vi "Header and Footer.vi"(4 "Header Footer Table Konfig":T8={"Header"={"Table Settings"={"Number of Columns"=2, "Width (%)"=100.0, "Relative Column Widths (%)"=[80.0, 20.0], "Horizontal Align"=0, "Header Rows"=0}, "Cell Defaults"={"Background Color"=16777215, "Horizontal Align"=3, "Vertical Align"=1, "Minimum Height"=0.0, "Fixed Height"=0.0, "Padding"={"Left"=2.0, "Top"=2.0, "Right"=2.0, "Bottom"=3.0}}, "Borders"={"Left"={"Enabled"=FALSE, "Width"=1.0, "Color"=0}, "Top"={"Enabled"=FALSE, "Width"=1.0, "Color"=0}, "Right"={"Enabled"=FALSE, "Width"=1.0, "Color"=0}, "Bottom"={"Enabled"=FALSE, "Width"=1.0, "Color"=0}, "Middle Horizontal"={"Enabled"=FALSE, "Width"=0.5, "Color"=0}, "Middle Vertical"={"Enabled"=FALSE, "Width"=0.5, "Color"=0}}}, "Footer"={"Table Settings"={"Number of Columns"=3, "Width (%)"=100.0, "Relative Column Widths (%)"=[15.0, 70.0, 15.0], "Horizontal Align"=0, "Header Rows"=0}, "Cell Defaults"={"Background Color"=16777215, "Horizontal Align"=0, "Vertical Align"=1, "Minimum Height"=0.0, "Fixed Height"=0.0, "Padding"={"Left"=2.0, "Top"=2.0, "Right"=2.0, "Bottom"=3.0}}, "Borders"={"Left"={"Enabled"=FALSE, "Width"=1.0, "Color"=0}, "Top"={"Enabled"=FALSE, "Width"=1.0, "Color"=0}, "Right"={"Enabled"=FALSE, "Width"=1.0, "Color"=0}, "Bottom"={"Enabled"=FALSE, "Width"=1.0, "Color"=0}, "Middle Horizontal"={"Enabled"=FALSE, "Width"=0.5, "Color"=0}, "Middle Vertical"={"Enabled"=FALSE, "Width"=0.5, "Color"=0}}}, "Footer Logo Row"={"Table Settings"={"Number of Columns"=1, "Width (%)"=100.0, "Relative Column Widths (%)"=[100.0], "Horizontal Align"=0, "Header Rows"=0}, "Cell Defaults"={"Background Color"=16777215, "Horizontal Align"=0, "Vertical Align"=1, "Minimum Height"=0.0, "Fixed Height"=0.0, "Padding"={"Left"=2.0, "Top"=2.0, "Right"=2.0, "Bottom"=3.0}}, "Borders"={"Left"={"Enabled"=FALSE, "Width"=1.0, "Color"=0}, "Top"={"Enabled"=FALSE, "Width"=1.0, "Color"=0}, "Right"={"Enabled"=FALSE, "Width"=1.0, "Color"=0}, "Bottom"={"Enabled"=FALSE, "Width"=1.0, "Color"=0}, "Middle Horizontal"={"Enabled"=FALSE, "Width"=0.5, "Color"=0}, "Middle Vertical"={"Enabled"=FALSE, "Width"=0.5, "Color"=0}}}} {"Footer Logo Row"."Cell Defaults"."Vertical Align" items=["Bottom", "Middle", "Top"]; "Footer Logo Row"."Cell Defaults"."Horizontal Align" items=["Center", "Justified", "JustifiedAll", "Left", "Right"]; "Footer Logo Row"."Table Settings"."Horizontal Align" items=["Center"=0, "Left"=3, "Right"=4]; "Footer"."Cell Defaults"."Vertical Align" items=["Bottom", "Middle", "Top"]; "Footer"."Cell Defaults"."Horizontal Align" items=["Center", "Justified", "JustifiedAll", "Left", "Right"]; "Footer"."Table Settings"."Horizontal Align" items=["Center"=0, "Left"=3, "Right"=4]; "Header"."Cell Defaults"."Vertical Align" items=["Bottom", "Middle", "Top"]; "Header"."Cell Defaults"."Horizontal Align" items=["Center", "Justified", "JustifiedAll", "Left", "Right"]; "Header"."Table Settings"."Horizontal Align" items=["Center"=0, "Left"=3, "Right"=4]}, 5 "Footer Image File Path":path, 6 "Font":T9={"Font"="Arial", "Size"=10, "Colour"=0, "Bold"=FALSE, "Italic"=FALSE, "Underline"=FALSE, "Strikethrough"=FALSE, "Font Encoding"=enum."Cp1252, WinANSI"}, 7 "Header Image File Path":path, 8 "error in":errorcluster, 9 "Header Footer OffsetCluster":T2={"Header Offset"=20.0, "Footer Offset"=120.0, "Margin"={"Left"=40.0, "Right"=40.0, "Top"=60.0, "Bottom"=160.0}}, 10 "Header Footer Text Cluster":T3={"Header Text"="Protokoll XYZ", "Footer Text"="IAG nG", "Time"="<TIMESTAMP>", "Page Number"="Page <P> of <PT>"}, 11 "Context In":refnum<class "Context.lvclass">=refnum) -> (0 "error out":errorcluster, 1 "Header Footer OffsetCluster out":T2={"Header Offset"=100.0, "Footer Offset"=300.0, "Margin"={"Left"=40.0, "Right"=40.0, "Top"=100.0, "Bottom"=300.0}}, 3 "Context out":refnum<class "Context.lvclass">)   [LabVIEW 2020, in "PDF Interface.lvlib" / "PDF Interface Helper.lvlib"]
doc: "Creates the custom header and footer layouts for the PDF test report."
uses:
  PDF Interface Helper.lvlib
  <vilib>/Simplicity AI/SAI_PDF_API/Classes/Context/Context.lvclass
  <vilib>/Simplicity AI/SAI_PDF_API/Classes/Context/Controls/SAI_PDF_Font.ctl
  <vilib>/Simplicity AI/SAI_PDF_API/Classes/Context/Controls/SAI_PDF_Font Encoding.ctl
  <vilib>/Simplicity AI/SAI_PDF_API/Classes/Table Builder/Controls/SAI_PDF_Table Configuration.ctl
  <vilib>/Simplicity AI/SAI_PDF_API/Classes/Table Builder/Controls/SAI_PDF_Table Horizontal Align.ctl
  <vilib>/Simplicity AI/SAI_PDF_API/Classes/Table Builder/Controls/SAI_PDF_Default Cell Format.ctl
  <vilib>/Simplicity AI/SAI_PDF_API/Classes/Table Builder/Controls/SAI_PDF_BorderLine.ctl
  <vilib>/Simplicity AI/SAI_PDF_API/Classes/Context/Controls/SAI_PDF_Margins.ctl
  <vilib>/Simplicity AI/SAI_PDF_API/Classes/Table Builder/Table Builder.lvclass
  PDF Interface.lvlib
panel:
  # "(Cp1252)"
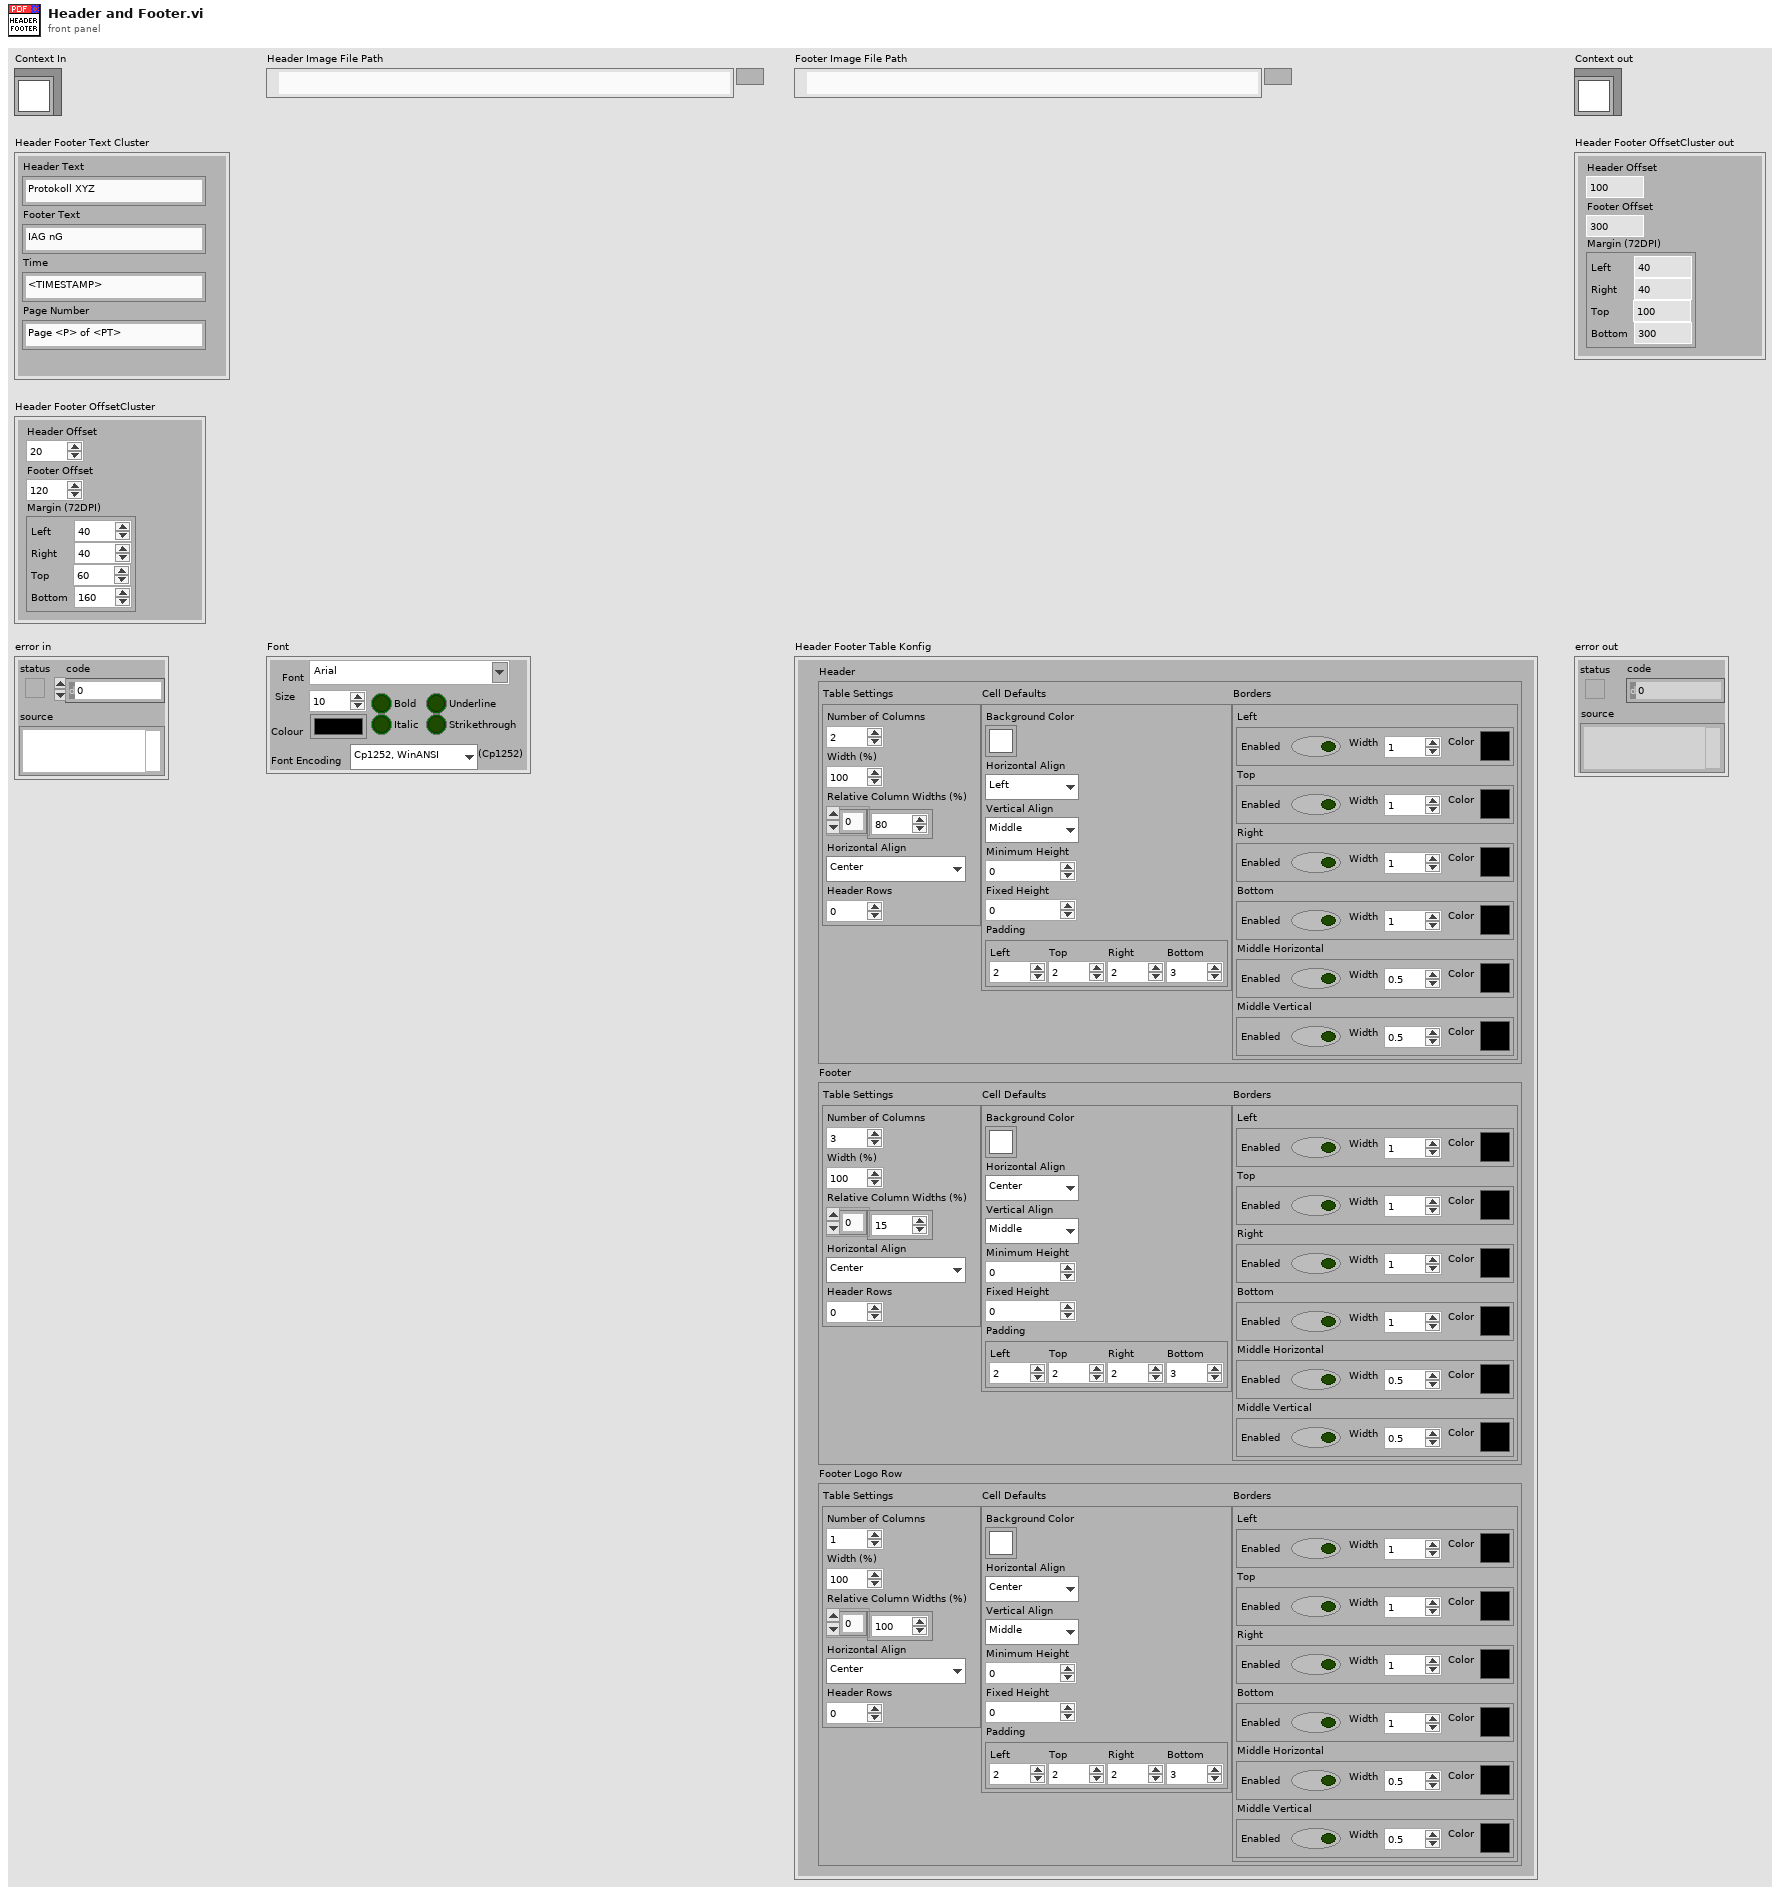
[diagram p1: front panel]
types:
  T1 = typedef "SAI_PDF_Toolkit.lvlib/Context.lvclass/SAI_PDF_Margins.ctl" = cluster{"Left":sgl, "Right":sgl, "Top":sgl, "Bottom":sgl}
  T2 = cluster{"Header Offset":sgl, "Footer Offset":sgl, "Margin":T1}
  T3 = cluster{"Header Text":string, "Footer Text":string, "Time":string, "Page Number":string}
  T4 = typedef "SAI_PDF_Toolkit.lvlib/Table Builder.lvclass/SAI_PDF_Table Configuration.ctl" = cluster{"Table Settings":cluster{"Number of Columns":i32, "Width (%)":sgl, "Relative Column Widths (%)":sgl[], "Horizontal Align":T5, "Header Rows":i32}, "Cell Defaults":T6, "Borders":cluster{"Left":T7, "Top":T7, "Right":T7, "Bottom":T7, "Middle Horizontal":T7, "Middle Vertical":T7}}
  T5 = typedef "SAI_PDF_Toolkit.lvlib/Table Builder.lvclass/SAI_PDF_Table Horizontal Align.ctl" = i32
  T6 = typedef "SAI_PDF_Toolkit.lvlib/Table Builder.lvclass/SAI_PDF_Default Cell Format.ctl" = cluster{"Background Color":u32, "Horizontal Align":i32, "Vertical Align":i32, "Minimum Height":sgl, "Fixed Height":sgl, "Padding":cluster{"Left":sgl, "Top":sgl, "Right":sgl, "Bottom":sgl}}
  T7 = typedef "SAI_PDF_Toolkit.lvlib/Table Builder.lvclass/SAI_PDF_BorderLine.ctl" = cluster{"Enabled":bool, "Width":sgl, "Color":u32}
  T8 = cluster{"Header":T4, "Footer":T4, "Footer Logo Row":T4}
  T9 = typedef "SAI_PDF_Toolkit.lvlib/Context.lvclass/SAI_PDF_Font.ctl" = cluster{"Font":string, "Size":i32, "Colour":u32, "Bold":bool, "Italic":bool, "Underline":bool, "Strikethrough":bool, "Font Encoding":T10}
  T10 = typedef "SAI_PDF_Toolkit.lvlib/Context.lvclass/SAI_PDF_Font Encoding.ctl" = enum16{"Cp1252, WinANSI", "IdentityH", "IdentityV", "Cp1250", "Cp1257", "MacRoman"}
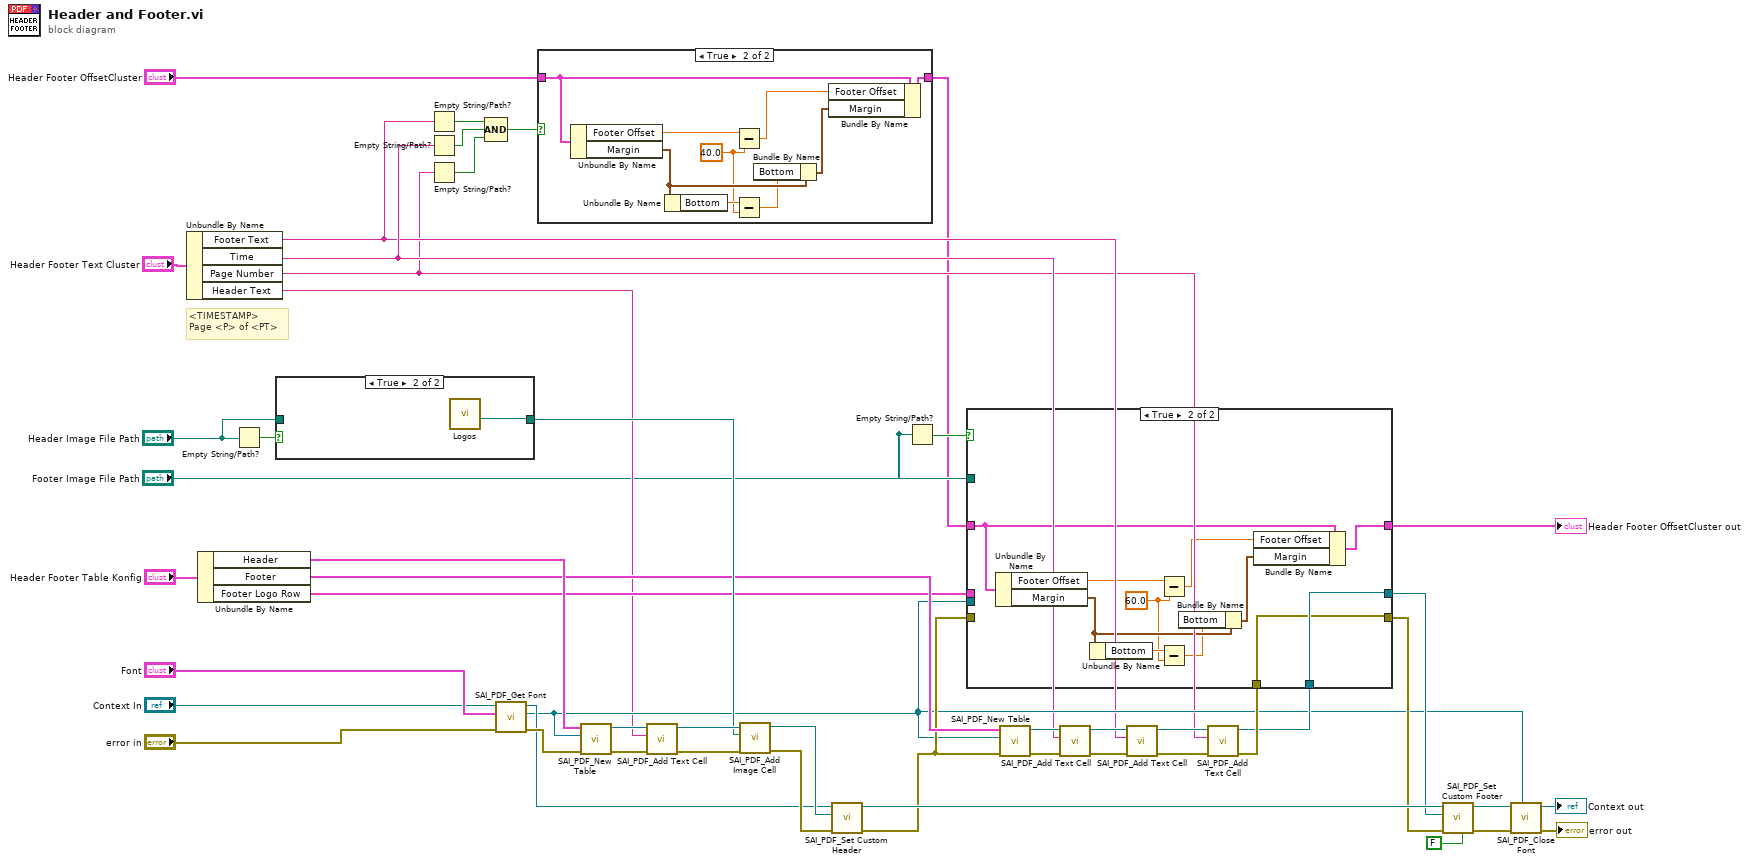
[diagram p0: block diagram]
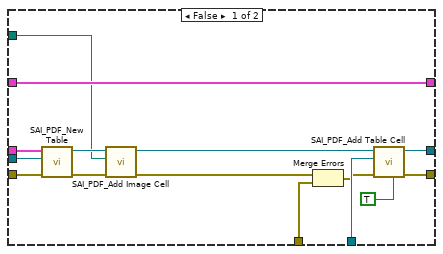
[diagram p3: hidden frame]
diagram:
  # "<TIMESTAMP>\nPage <P> of <PT>"
  n1 = Unbundle By Name("Header Footer Text Cluster") -> ("Footer Text"=w8:string, "Time"=w9:string, "Page Number"=w7:string, "Header Text"=w13:string)
  n2 = Unbundle By Name("Header Footer Table Konfig") -> ("Header"=w27:T4, "Footer"=w26:T4, "Footer Logo Row"=w25:T4)
  n3 = Empty String/Path?(string/path="Header Image File Path") -> (empty?=w33:bool)
  n4 = case shown="True" w33 {
    tunnel: [w51 w52] -> w32
    tunnel: "Header Image File Path" -> [w51 _]
    frame False {
    }
    frame True {
      n5 = call "Logos.vi"() -> ("Default  Header Image File Path"=w52:path)  [unwired: 8 in, 3 out]
    }
  }
  n6 = Empty String/Path?(string/path=w8) -> (empty?=w6:bool)
  n7 = Empty String/Path?(string/path=w9) -> (empty?=w5:bool)
  n8 = Empty String/Path?(string/path=w7) -> (empty?=w4:bool)
  n9 = Compound Arithmetic op=AND ("Mehrfacharithmetik")(w6, w5, w4) -> (w3:bool)
  n10 = call <vilib>:"SAI_PDF_Get Font.vi"("error in"="error in", "Font"="Font", "Context In"="Context In") -> ("error out"=w50:errorcluster, "Font"=w18:refnum<class "Font.lvclass">, "Context Out"=w43:refnum<class "Context.lvclass">)  [unwired: 6 out]
  n11 = case shown="True" w3 {
    tunnel: "Header Footer OffsetCluster" -> [w53 w55]
    tunnel: [w53 w54] -> w1
    frame False {
    }
    frame True {
      w56 = sgl 40.0 ("y")
      n12 = Unbundle By Name(w55) -> ("Footer Offset"=w62:sgl, "Margin"=w60:T1)
      n13 = Unbundle By Name(w60) -> ("Bottom"=w58:sgl)
      n14 = Subtract(x=w62, y=w56) -> (x-y=w61:sgl)
      n15 = Subtract(x=w58, y=w56) -> (x-y=w57:sgl)
      n16 = Bundle By Name(cluster=w60, "Bottom"=w57) -> (w59:T1)
      n17 = Bundle By Name(cluster=w55, "Footer Offset"=w61, "Margin"=w59) -> (w54:T2)
    }
  }
  n18 = call <vilib>:"SAI_PDF_New Table.vi"("error in"=w50, "Font In"=w18, "Table Configuration"=w27) -> ("error out"=w47:errorcluster, "Table Builder"=w46:refnum<class "Table Builder.lvclass">)  [unwired: 7 out]
  n19 = call <vilib>:"SAI_PDF_Add Text Cell.vi"("error in"=w47, "Text"=w13, "Table Builder In"=w46) -> ("error out"=w49:errorcluster, "Table Builder Out"=w48:refnum<class "Table Builder.lvclass">)  [unwired: 1 in, 6 out]
  n20 = call <vilib>:"SAI_PDF_Add Image Cell.vi"("error in"=w49, "Image File Path"=w32, "Table Builder In"=w48) -> ("error out"=w45:errorcluster, "Table Builder Out"=w44:refnum<class "Table Builder.lvclass">)  [unwired: 3 in, 4 out]
  n21 = call <vilib>:"SAI_PDF_Set Custom Header.vi"("error in"=w45, "Table In"=w44, "Context In"=w43) -> ("error out"=w24:errorcluster, "Context Out"=w35:refnum<class "Context.lvclass">)  [unwired: 7 out]
  n22 = Empty String/Path?(string/path="Footer Image File Path") -> (empty?=w12:bool)
  n23 = call <vilib>:"SAI_PDF_New Table.vi"("error in"=w24, "Font In"=w18, "Table Configuration"=w26) -> ("error out"=w29:errorcluster, "Table Builder"=w30:refnum<class "Table Builder.lvclass">)  [unwired: 7 out]
  n24 = call <vilib>:"SAI_PDF_Add Text Cell.vi"("error in"=w29, "Text"=w9, "Table Builder In"=w30) -> ("error out"=w39:errorcluster, "Table Builder Out"=w38:refnum<class "Table Builder.lvclass">)  [unwired: 1 in, 6 out]
  n25 = call <vilib>:"SAI_PDF_Add Text Cell.vi"("error in"=w39, "Text"=w8, "Table Builder In"=w38) -> ("error out"=w34:errorcluster, "Table Builder Out"=w36:refnum<class "Table Builder.lvclass">)  [unwired: 1 in, 6 out]
  n26 = call <vilib>:"SAI_PDF_Add Text Cell.vi"("error in"=w34, "Text"=w7, "Table Builder In"=w36) -> ("error out"=w37:errorcluster, "Table Builder Out"=w23:refnum<class "Table Builder.lvclass">)  [unwired: 1 in, 6 out]
  n27 = case shown="True" w12 {
    tunnel: w37 -> [w77 w87]
    tunnel: w25 -> [w75 _]
    tunnel: w24 -> [w74 _]
    tunnel: w23 -> [w70 w88]
    tunnel: [w69 w88] -> w22
    tunnel: [w66 w87] -> w21
    tunnel: w18 -> [w65 _]
    tunnel: w1 -> [w64 w86]
    tunnel: [w64 w85] -> w11
    tunnel: "Footer Image File Path" -> [w63 _]
    frame False {
      n28 = call <vilib>:"SAI_PDF_New Table.vi"("error in"=w74, "Font In"=w65, "Table Configuration"=w75) -> ("error out"=w72:errorcluster, "Table Builder"=w73:refnum<class "Table Builder.lvclass">)  [unwired: 7 out]
      n29 = call <vilib>:"SAI_PDF_Add Image Cell.vi"("error in"=w72, "Image File Path"=w63, "Table Builder In"=w73) -> ("error out"=w68:errorcluster, "Table Builder Out"=w71:refnum<class "Table Builder.lvclass">)  [unwired: 3 in, 4 out]
      n30 = Merge Errors(w68, w77) -> (w67:errorcluster)
      n31 = call <vilib>:"SAI_PDF_Add Table Cell.vi"("Close References (f)"=TRUE, "error in"=w67, "Cell Table Builder In"=w70, "Table Builder In"=w71) -> ("error out"=w66:errorcluster, "Table Builder Out"=w69:refnum<class "Table Builder.lvclass">)  [unwired: 1 in, 5 out]
    }
    frame True {
      w78 = sgl 60.0 ("y")
      n32 = Unbundle By Name(w86) -> ("Footer Offset"=w84:sgl, "Margin"=w82:T1)
      n33 = Unbundle By Name(w82) -> ("Bottom"=w80:sgl)
      n34 = Subtract(x=w84, y=w78) -> (x-y=w83:sgl)
      n35 = Subtract(x=w80, y=w78) -> (x-y=w79:sgl)
      n36 = Bundle By Name(cluster=w82, "Bottom"=w79) -> (w81:T1)
      n37 = Bundle By Name(cluster=w86, "Footer Offset"=w83, "Margin"=w81) -> (w85:T2)
    }
  }
  "Header Footer OffsetCluster out" <- w11
  n38 = call <vilib>:"SAI_PDF_Set Custom Footer.vi"("Close References (f)"=FALSE, "error in"=w21, "Table In"=w22, "Context In"=w35) -> ("error out"=w19:errorcluster, "Context Out"=w20:refnum<class "Context.lvclass">)  [unwired: 6 out]
  n39 = call <vilib>:"SAI_PDF_Close Font.vi"("Font"=w18, "error in"=w19, "Context In"=w20) -> ("error out"=→"error out":errorcluster, "Context Out"=→"Context out":refnum<class "Context.lvclass">)  [unwired: 7 out]
